vi "IniFindParam (SubVI).vi"(10 "Array":string[][](array[string]), 11 "element":string) -> (3 "StringOut":string)   [LabVIEW 2017, in "LV_Unicorn.lvlib"]
uses:
  LV_Unicorn.lvlib
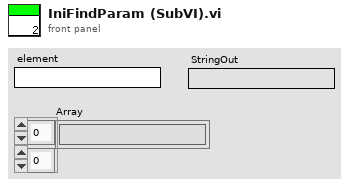
[diagram p1: front panel]
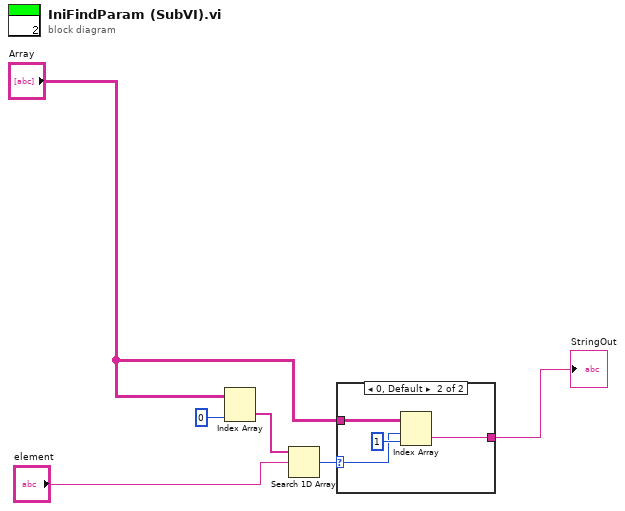
[diagram p0: block diagram]
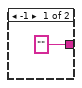
[diagram p2: hidden frame]
diagram:
  n1 = Index Array(array="Array", index (col)=0 ("disabled index (col)")) -> (element=w3:string[])  [unwired: 1 in]
  n2 = Search 1D Array(1D array=w3, element="element") -> (index of element=w6:i32)  [unwired: 1 in]
  n3 = case shown="0, Default" w6 {
    selector: w6 -> [_ w9]
    tunnel: "Array" -> [_ w11]
    tunnel: ["" ("StringOut") w8] -> w1
    frame -1 {
    }
    frame 0, Default {
      n4 = Index Array(array=w11, index (row)=w9, index (col)=1 ("disabled index (col)")) -> (element=w8:string)
    }
  }
  "StringOut" <- w1
